vi "Morse to Boolean.vi"(11 "Morse Code Array":string[](array[string])) -> (3 "Boolean Array":bool[](array[boolean]))   [LabVIEW 2022 SP3]
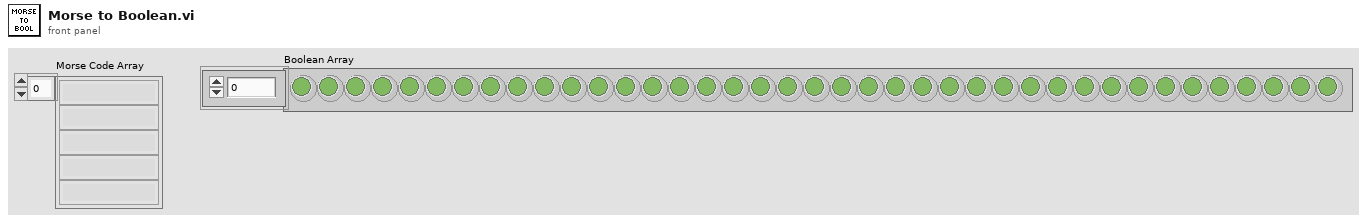
[diagram p1: front panel]
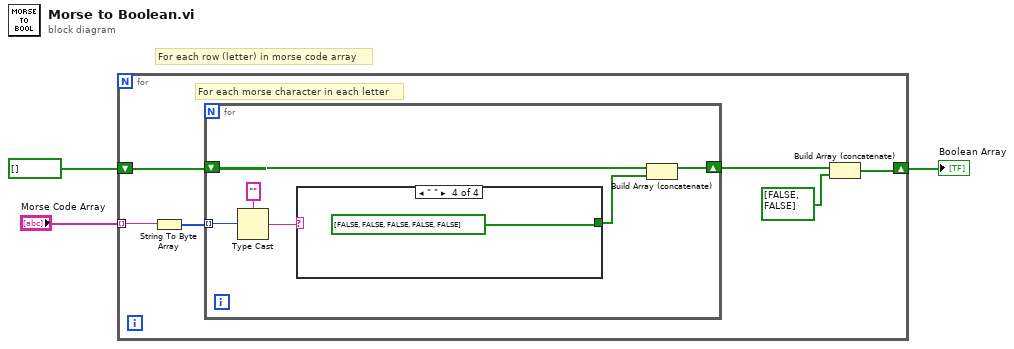
[diagram p0: block diagram]
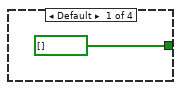
[diagram p2: hidden frame]
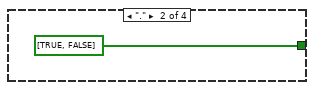
[diagram p3: hidden frame]
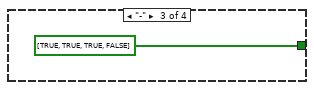
[diagram p4: hidden frame]
diagram:
  # "For each row (letter) in morse code array"
  n1 = for {
    tunnel: "Morse Code Array" -> [w4] mode=indexing
    shift-right: [w7] -> w2
    shift-left: bool[] [] -> [w9]
    # "For each morse character in each letter"
    n2 = String To Byte Array(string=w4) -> (unsigned byte array=w5:u8[])
    n3 = for {
      shift-right: [w13] -> w8
      shift-left: w9 -> [w14]
      tunnel: w5 -> [w12] mode=indexing
      n4 = Type Cast(type="", x=w12) -> (*(type *) &x=w11:string)
      n5 = case shown="\" \"" w11 {
        tunnel: [bool[] [] bool[] [TRUE, FALSE] bool[] [TRUE, TRUE, TRUE, FALSE] bool[] [FALSE, FALSE, FALSE, FALSE, FALSE]] -> w15
        frame Default {
        }
        frame "." {
        }
        frame "-" {
        }
        frame " " {
        }
      }
      n6 = Build Array (concatenate)(w14, w15) -> (w13:bool[])
    }
    n7 = Build Array (concatenate)(w8, bool[] [FALSE, FALSE] ("array")) -> (w7:bool[])
  }
  "Boolean Array" <- w2
